vi "Row-Column Average for 2D array LV2016 NIVerified.vi"() -> ()   [LabVIEW 2016]
uses:
  <vilib>/Analysis/baseanly.llb/Mean (DBL).vi
  <vilib>/Analysis/NI_AALBase.lvlib
panel:
  out "Total Array Average":dbl
  out "Column Averages":dbl[](array[numeric])
  out "Row Averages":dbl[](array[numeric])
  in  "2D Array":dbl[][](array[numeric])
  # "Overview:\nThis example shows how you can calculate row and column averages for a 2D array.\nRequirements:\nLabVIEW 2009 (or compatible)\nInstructions:\n1.Fill the table with  digits\n2.Run"
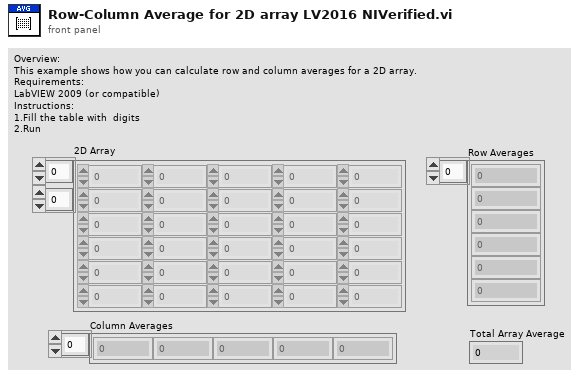
[diagram p1: front panel]
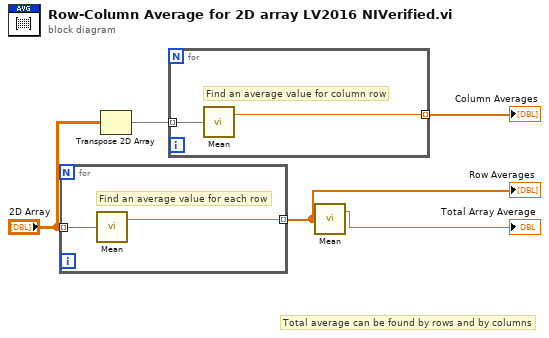
[diagram p0: block diagram]
diagram:
  # "Total average can be found by rows and by columns"
  n1 = for {
    tunnel: "2D Array" -> [w7] mode=indexing
    tunnel: [w6] -> w2 mode=indexing
    # "Find an average value for each row"
    n2 = call-poly <vilib>:"Mean.vi"("X"=w7) -> ("mean"=w6:dbl)  [unwired: 1 out]
  }
  "Row Averages" <- w2
  n3 = Transpose 2D Array(2D array="2D Array") -> (transposed array=w5:dbl[][])
  n4 = for {
    tunnel: w5 -> [w9] mode=indexing
    tunnel: [w8] -> w1 mode=indexing
    # "Find an average value for column row"
    n5 = call-poly <vilib>:"Mean.vi"("X"=w9) -> ("mean"=w8:dbl)  [unwired: 1 out]
  }
  "Column Averages" <- w1
  n6 = call-poly <vilib>:"Mean.vi"("X"=w2) -> ("mean"=→"Total Array Average":dbl)  [unwired: 1 out]
